vi "Launcher.vi"   [LabVIEW 2024]
uses:
  src/Error Reporting Actor/Error Reporter/Error Reporter/Error Reporter.lvclass
  Sample Error Reporter/Sample Error Reporter/Sample Error Reporter.lvclass
  Sample Error Manager/Sample Error Manager/Sample Error Manager.lvclass
  C:/Users/uspoaotto/OneDrive - Oregon Tool/Desktop/working copies/errorReportingActor/src/Error Reporting Actor/Error Reporter/Error Reporter/Error Reporter.lvclass
  C:/Program Files (x86)/National Instruments/LabVIEW 2024/vi.lib/ActorFramework/Actor/Actor.lvclass
  C:/Users/uspoaotto/OneDrive - Oregon Tool/Desktop/working copies/errorReportingActor/samples/Sample Error Reporter/Sample Error Reporter/Sample Error Reporter.lvclass
  C:/Users/uspoaotto/OneDrive - Oregon Tool/Desktop/working copies/errorReportingActor/src/Error Reporting Actor/Error Manager/Error Manager/Error Manager.lvclass
  C:/Users/uspoaotto/OneDrive - Oregon Tool/Desktop/working copies/errorReportingActor/src/Error Reporting Actor/~Error/~Error/~Error.lvclass
  C:/Users/uspoaotto/OneDrive - Oregon Tool/Desktop/working copies/errorReportingActor/samples/Sample Error Manager/Sample Error Manager/Sample Error Manager.lvclass
panel:
  # "LAUNCHER"
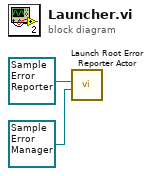
[diagram p0: block diagram]
diagram:
  n1 = call "Launch Root Error Reporter Actor.vi"("Error Manager in"=refnum<class "Sample Error Manager.lvclass"> refnum ("Sample Error Manager.lvlib:Sample Error Manager.lvclass"), "Error Reporter in"=refnum<class "Sample Error Reporter.lvclass"> refnum ("Sample Error Reporter.lvlib:Sample Error Reporter.lvclass")) -> ()  [unwired: 8 in, 2 out]
